vi "set_data.vi"(7 "LabVIEW Web Service Request":refnum<class "Web Request.lvclass">) -> ()   [LabVIEW 2014]
uses:
  <vilib>/wsapi/Web Request.lvclass
  DataManager/StateStore/Controls/DataFunction.ctl
panel:
  # "Use the Web Service Request input terminal to call the VIs on the Web Services palette. Do not remove it from the connector pane unless you don't need access to the palette."
  # "Each additional control wired to the connector pane will be available as an input in the URL. To include an indicator in terminal-mode output (the default setting), it must also be wired to the connector pane."
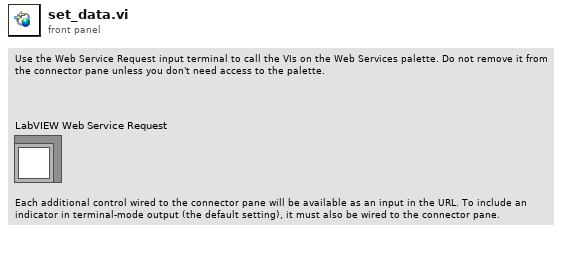
[diagram p1: front panel]
types:
  T1 = cluster{"train_control_array":cluster{"uuid":string, "throttle":dbl, "brake":dbl, "horn":dbl, "wait":dbl, "name":string, "mode":string, "dest":string}[], "switch_control_array":cluster{"switch_posit":cluster{"x":dbl, "y":dbl, "z":dbl}, "switch":bool, "invert":bool, "wait":dbl}[]}
  T2 = typedef "DataFunction.ctl" = enum16{"Initialise", "Release", "Get Data", "Set Data", "Preview Data"}
  T3 = cluster{"uuid":string, "throttle":dbl, "brake":dbl, "horn":dbl, "wait":dbl, "name":string, "mode":string, "dest":string}[]
  T4 = typedef "CData Core Control.ctl" = cluster{"train_data_array":cluster{"uuid":string, "int":i32, "posit_array":cluster{"x":dbl, "y":dbl, "z":dbl}[]}[], "train_control_array":cluster{"uuid":string, "throttle":dbl, "brake":dbl, "horn":dbl, "wait":dbl, "name":string, "mode":string, "dest":string}[], "switch_data_array":cluster{"switch_posit":cluster{"x":dbl, "y":dbl, "z":dbl}, "manual":bool}[], "switch_control_array":cluster{"switch_posit":cluster{"x":dbl, "y":dbl, "z":dbl}, "switch":bool, "invert":bool, "wait":dbl}[]}
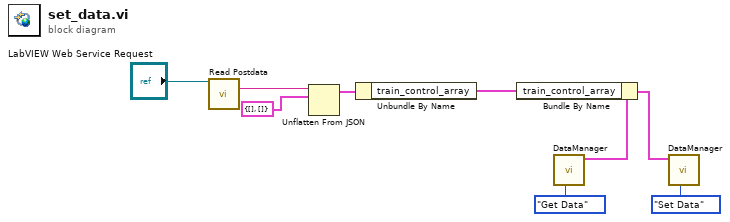
[diagram p0: block diagram]
diagram:
  n1 = call <vilib>:"Read Postdata.vi"("LabVIEW Web Service Request"="LabVIEW Web Service Request") -> ("postdata"=w5:string)  [unwired: 12 in, 2 out]
  n2 = Unflatten From JSON(JSON string=w5, type and defaults=T1 {"train_control_array"=[], "switch_control_array"=[]} ("output cluster")) -> (value=w2:T1)  [unwired: 5 in, 1 out]
  n3 = Unbundle By Name(w2) -> ("train_control_array"=w1:T3)
  n4 = call "DataManager.vi"("DataFunction"=DataFunction."Get Data") -> ("CData Out"=w4:T4)  [unwired: 9 in, 1 out]
  n5 = Bundle By Name(cluster=w4, "train_control_array"=w1) -> (w7:T4)
  n6 = call "DataManager.vi"("DataFunction"=DataFunction."Set Data", "CData In"=w7) -> ()  [unwired: 8 in, 2 out]
